vi "Multirate FIR Filter.vi"() -> ()   [LabVIEW 2023]
doc: "This VI illustrates the use of Stream Channels to create a multi-stage multi-rate FIR resampling filter."
uses:
  <extravilib>/ChannelInstances/Stream-dbl/Read With Abort.vi
  <extravilib>/ChannelInstances/Stream-dbl/Write With Abort.vi
  <extravilib>/ChannelInstances/Stream-dbl/EndpointRead.vi
  <extravilib>/ChannelInstances/Stream-dbl/Endpoint.vi
  <extravilib>/ChannelInstances/Stream-dbl/Instantiate.vi
  <extravilib>/ChannelInstances/Stream-dbl/)Channel.vi
  <resource>/ChannelSupport/_ChannelSupport/WaitIfNeeded.vi
  <extravilib>/ChannelInstances/Stream-dbl.lvlib
panel:
  in  "gain":dbl(slide)=1.0 scale=0.0..2.0
  in  "Stop":bool
  in  "frequency":dbl(knob)=5.0 scale=0.0..10.0 scale format="%.1f"
  out "Output Signal":dbl(graph)
  out "Input Signal":dbl(graph)
  # "Overview: Demonstrates the use of the Stream Channel in making a multi-stage multi-rate FIR filter for resampling an audio waveform.\n\nInstructions:\nRun the VI.  Observe the input data.  Observe the delayed output data to be the same as the input but sampled at a slightly higher rate.  Adjust gain and frequency to vary the signal."
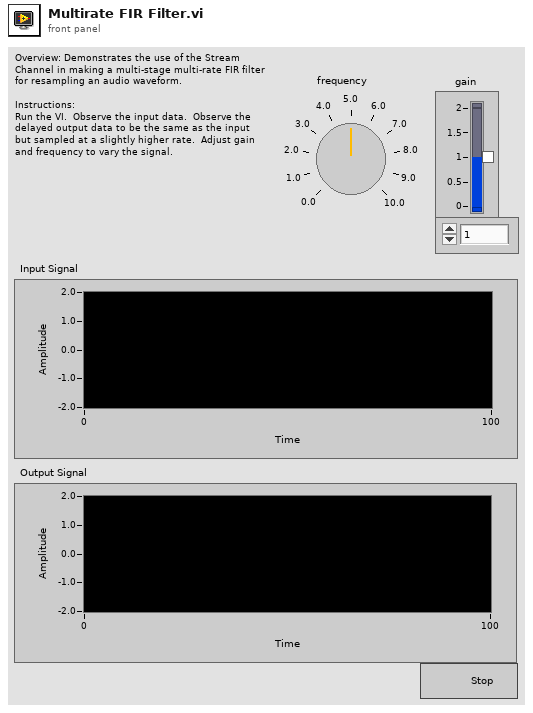
[diagram p1: front panel]
types:
  T1 = typedef "Stream-dbl.lvlib/)Channel.ctl" = refnum<queue>
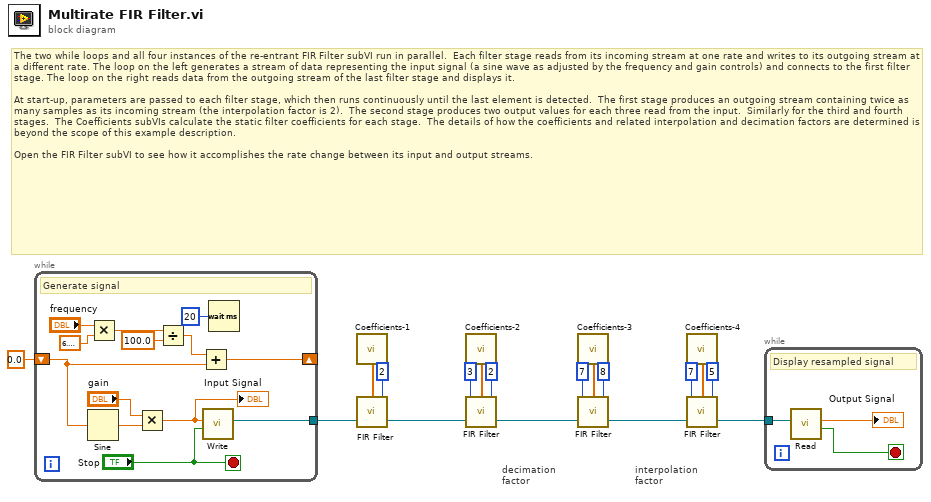
[diagram p0: block diagram]
diagram:
  # "The two while loops and all four instances of the re-entrant FIR Filter subVI run in parallel.  Each filter stage reads from its incoming stream at one rate and writes to its outgoing stream at a different rate. The loop on the left generates a stream of data representing the input signal (a sine wave as adjusted by the frequency and gain controls) and connects to the first filter stage. The loop on the right reads data from the outgoing stream of the last filter stage and displays it.\n\nAt start-up, parameters are passed to each filter stage, which then runs continuously until the last element is detected.  The first stage produces an outgoing stream containing twice as many samples as its incoming stream (the interpolation factor is 2).  The second stage produces two output values for each three read from the input.  Similarly for the third and fourth stages.  The Coefficients subVIs calculate the static filter coefficients for each stage.  The details of how the coefficients and related interpolation and decimation factors are determined is beyond the scope of this example description.\n\nOpen the FIR Filter subVI to see how it accomplishes the rate change between its input and output streams."
  # "interpolation\nfactor"
  # "decimation\nfactor"
  n1 = while {
    shift-right: [w28] -> _
    shift-left: 0.0 -> [w29]
    tunnel: [w19] -> w5
    stop <- "Stop" stop-if-true
    # "Generate signal"
    n2 = Sine(x=w29) -> (sin(x)=w22:dbl)
    n3 = Multiply(x="frequency", y=6.283185307179586) -> (x*y=w25:dbl)
    n4 = Multiply(x="gain", y=w22) -> (x*y=w20:dbl)
    "Input Signal" <- w20
    n5 = Divide(x=w25, y=100.0) -> (x/y=w24:dbl)
    n6 = Add(x=w24, y=w29) -> (x+y=w28:dbl)
    n7 = call <extravilib>:"Write.vi"("last element? (F)"="Stop", "element"=w20) -> ("channel"=w19:T1)  [unwired: 7 in, 2 out]
    n8 = Wait (ms)(milliseconds to wait=u32 20 ("millisecond multiple")) -> ()  [unwired: 1 out]
  }
  n9 = call "Coefficients-1.vi"() -> ("filter coefficients"=w10:dbl[])
  n10 = call "FIR Filter.vi"("stream in"=w5, "filter coefficients"=w10, "interpolation factor (1)"=2) -> ("stream out"=w1:T1)  [unwired: 1 in]
  n11 = call "Coefficients-2.vi"() -> ("filter coefficients"=w9:dbl[])
  n12 = call "FIR Filter.vi"("stream in"=w1, "decimation factor (1)"=3, "filter coefficients"=w9, "interpolation factor (1)"=2) -> ("stream out"=w4:T1)
  n13 = call "Coefficients-3.vi"() -> ("filter coefficients"=w8:dbl[])
  n14 = call "FIR Filter.vi"("stream in"=w4, "decimation factor (1)"=7, "filter coefficients"=w8, "interpolation factor (1)"=8) -> ("stream out"=w3:T1)
  n15 = call "Coefficients-4.vi"() -> ("filter coefficients"=w7:dbl[])
  n16 = call "FIR Filter.vi"("stream in"=w3, "decimation factor (1)"=7, "filter coefficients"=w7, "interpolation factor (1)"=5) -> ("stream out"=w2:T1)
  n17 = while {
    tunnel: w2 -> [w33]
    stop <- w31 stop-if-true
    # "Display resampled signal"
    n18 = call <extravilib>:"Read.vi"("channel"=w33) -> ("last element?"=w31:bool, "element"=→"Output Signal":dbl)  [unwired: 6 in, 3 out]
  }
